vi "APIBiasDiffupdate.vi"(8 "Error In":errorcluster, 11 "Data":variant) -> (0 "Error Out":errorcluster)   [LabVIEW 2023, in "QSM - Main.lvlib"]
uses:
  QSM - Main.lvlib
  Controls/Message Queue Element Position.ctl
  Controls/State Machine Message.ctl
  SubVIs/Enqueue Message (Single).vi
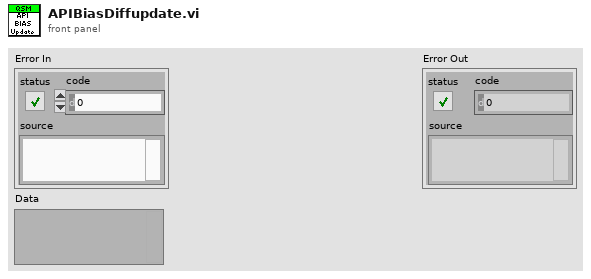
[diagram p1: front panel]
types:
  T1 = typedef "QSM - Main.lvlib/State Machine Message.ctl" = enum16{"Initialize", "Operator Signon", "Editor", "Security", "Select Tube", "Select Sched", "View Sched", "View IO/DOCS", "New Gx Val", "View LIMITS", "View ALARMS", "Start Step Change", "New Serial Number", "RUN Initiated", "RESET Initiated", "PLC Step Change", "PROC OK CHECK", "PROC NOK", "APIProcNOKUpdate", "APILimitUpdate", "APIOperatorUpdate", "APIAnalogIOUpdate", "APIOffsetGainUpdate", "APIGXValsUpdate", "APIBiasDiffUpdate", "ALARM CHECK", "ALARM ACTIVE", "CHECKS", "BIAS ZER", "DIFF ZER", "DIFF TOGGLE", "Handle Error", "Exit"}
  T2 = typedef "QSM - Main.lvlib/Message Queue Element Position.ctl" = enum16{"Front", "Back"}
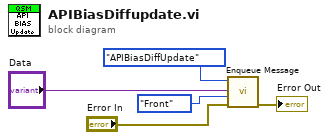
[diagram p0: block diagram]
diagram:
  n1 = call-poly "Enqueue Message.vi"("Error In"="Error In", "Message Position"=Message_Queue_Element_Position."Front", "Data"="Data", "State Machine Message"=State_Machine_Message."APIBiasDiffUpdate") -> ("Error Out"=→"Error Out":errorcluster)  [unwired: 7 in]
